vi "Read.vi"(11 "Setup in":refnum<class "Setup.lvclass">) -> (2 "Setup":T1)   [LabVIEW 2025, in "jettl.lvlib" / "Setup.lvlib" / "Setup.lvclass"]
uses:
  Setup.lvclass
  Attributes/Attributes/Attributes.lvclass
  Msg/Msg.lvclass
  Actor/Msg Set.ctl
  Actor/Actor.lvlib
  Transport/Transport/Transport.lvclass
  Setup.ctl
  Setup.lvlib
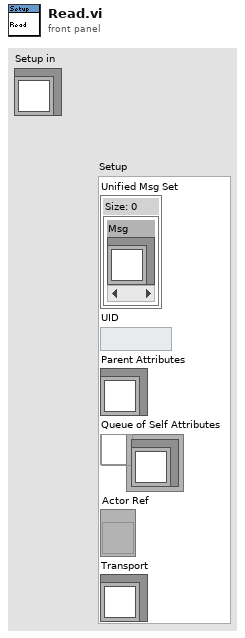
[diagram p1: front panel]
types:
  T1 = typedef "jettl.lvlib/Setup.lvlib/Setup.ctl" = cluster{"Unified Msg Set":T2, "UID":string, "Parent Attributes":refnum<class "Attributes.lvclass">, "Queue of Self Attributes":refnum<queue>, "Actor Ref":refnum<vi>, "Transport":refnum<class "Transport.lvclass">}
  T2 = typedef "jettl.lvlib/Actor.lvlib/Msg Set.ctl" = set{refnum<class "Msg.lvclass">}
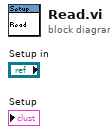
[diagram p0: block diagram]
diagram:
